vi "statistics-deviation.vi"() -> ()   [LabVIEW 2015]
uses:
  globalVarSD.vi
  <vilib>/Analysis/NI_AALBase.lvlib
panel:
  out "éléments":dbl[](array[numeric])
  out "OD":T1(graph)
  out "SC":cluster{"wavelengths":dbl[], "Tableau":dbl[]}[](graph)
  in  "number of aq":i32=1
  in  "wavelength":dbl=400.0
  out "stadard dev":dbl(slide) scale=0.0..0.005 scale format="%#_6e"
  out "mean":dbl format="%0.1e"
  in  "stop":bool
  in  "max queue size":i32=20
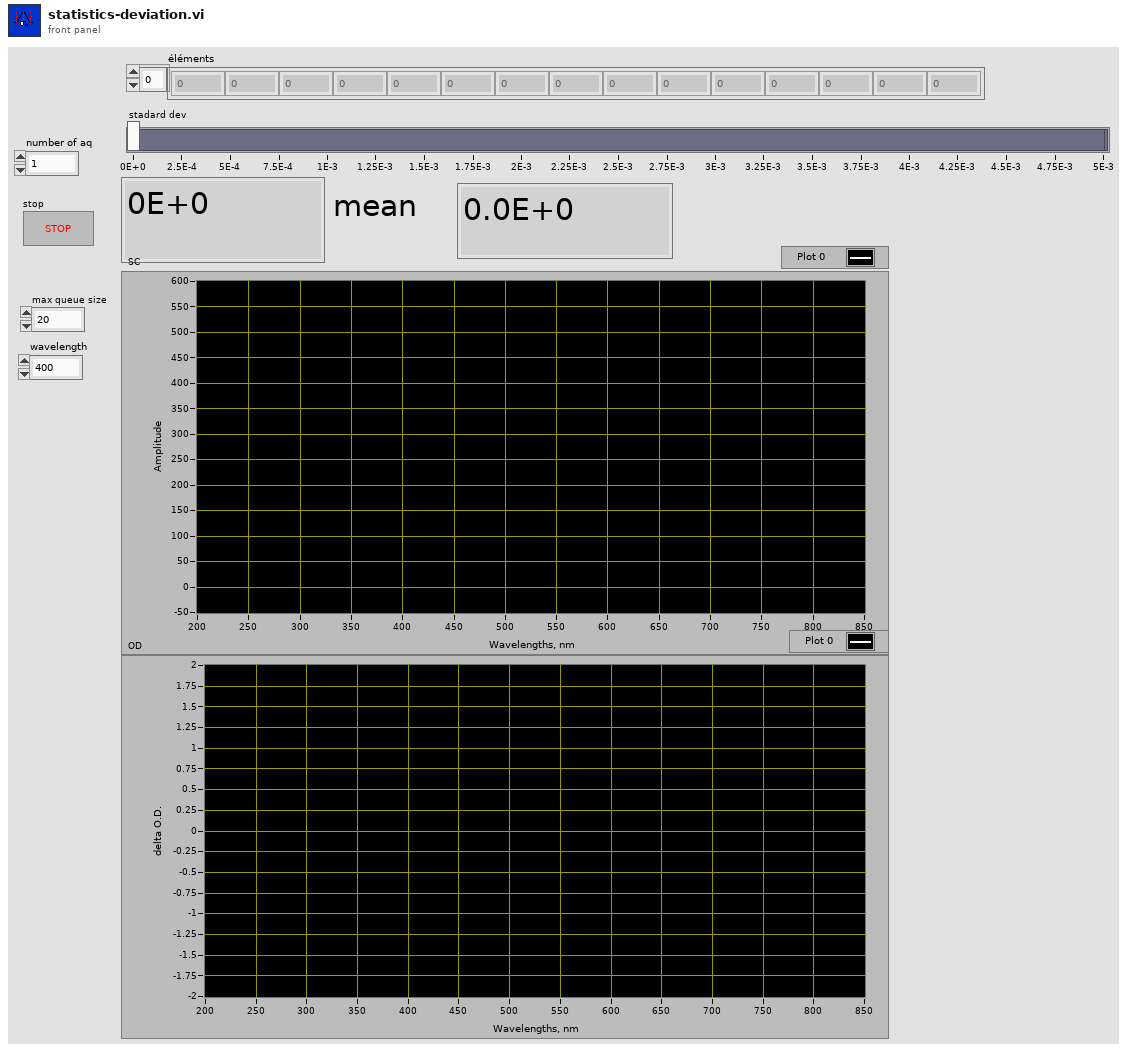
[diagram p1: front panel]
types:
  T1 = cluster{"wavelengths":dbl[], "-log(x)=log(1/x)":dbl[]}
  T2 = typedef "data-cluster.ctl" = cluster{"BG":i32[], "Ie":i32[], "I0":i32[]}[]
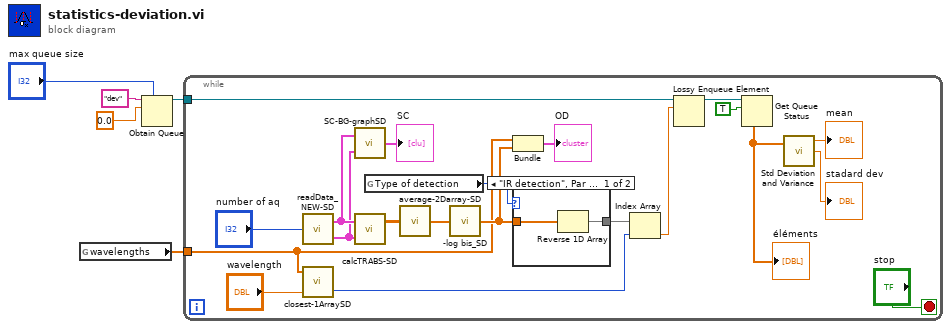
[diagram p0: block diagram]
diagram:
  n1 = global read "globalVarSD.vi" "wavelengths"() -> (w1:dbl[])
  n2 = Obtain Queue(max queue size (-1, unlimited)="max queue size", name (unnamed)="dev", element data type=0.0 ("y")) -> (queue out=w2:refnum<queue>)  [unwired: 2 in, 2 out]
  n3 = while {
    tunnel: w2 -> [w24]
    tunnel: w1 -> [w7]
    stop <- "stop" stop-if-true
    n4 = call "readData_NEW-SD.vi"("number of aq"="number of aq") -> ("I channel seq"=w11:T2, "II channel seq"=w10:T2)
    n5 = call "closest-1ArraySD.vi"("desired element"="wavelength", "1D Array"=w7) -> ("closest index"=w13:i32)  [unwired: 1 in, 1 out]
    n6 = call "SC-BG-graphSD.vi"("II channel seq"=w10, "I channel seq"=w11) -> ("Array"=→"SC":cluster{"wavelengths":dbl[], "Tableau":dbl[]}[])
    n7 = call "calcTRABS-SD.vi"("II channel seq"=w10, "I channel seq"=w11) -> ("TRanS multiple measurements"=w15:dbl[][])  [unwired: 1 out]
    n8 = global read "globalVarSD.vi" "Type of detection"() -> (w17:enum32{"IR detection", "UV-vis detection"})
    n9 = call "average-2Darray-SD.vi"("2D array"=w15) -> ("out array"=w16:dbl[])
    n10 = call "-log bis_SD.vi"("Transmission"=w16) -> ("-log(x)=log(1/x)"=w8:dbl[])
    n11 = Bundle("wavelengths"=w7, "-log(x)=log(1/x)"=w8) -> (→"OD":T1)  [unwired: 1 in]
    n12 = case shown="\"IR detection\", Par défaut" w17 {
      tunnel: w8 -> [w28 w29]
      tunnel: [w27 w29] -> w18
      frame "IR detection", Default {
        n13 = Reverse 1D Array(array=w28) -> (reversed array=w27:dbl[])
      }
      frame "UV-vis detection" {
      }
    }
    n14 = Index Array(array=w18, index=w13) -> (element=w12:dbl)
    n15 = Lossy Enqueue Element(queue=w24, element=w12) -> (queue out=w23:refnum<queue>)  [unwired: 1 in, 3 out]
    n16 = Get Queue Status(queue=w23, return elements? (F)=TRUE) -> (elements=w22:dbl[])  [unwired: 1 in, 7 out]
    "éléments" <- w22
    n17 = call <vilib>:"Std Deviation and Variance.vi"("X"=w22) -> ("mean"=→"mean":dbl, "standard deviation"=→"stadard dev":dbl)  [unwired: 1 in, 1 out]
  }
